vi "ziExample-HF2-RTK-PI.vi"() -> ()   [LabVIEW 2009]
doc: "This is an example for a Zurich Instruments HF2 instrument with RTK option installed. \nThis VI works together with a program for the real-time processor to implement two PI (Proportional-Integral) controllers. The controllers themselves run on the real-time processor. This VI communicates with the real-time processor to configure the controllers.\nThe program for the real-time processor is implemented in the file Main.c."
uses:
  <instrlib>/Zurich Instruments LabOne/Public/Configure/ziGetValueString.vi
  <instrlib>/Zurich Instruments LabOne/Zurich Instruments LabOne.lvlib
panel:
  in  "pid2_invert":bool
  in  "pid1_invert":bool
  in  "pid2_input_select2":enum16{"X", "Y", "R", "Theta"}(ring) caption="Signal"
  in  "pid1_input_select2":enum16{"X", "Y", "R", "Theta"}(ring) caption="Signal"
  in  "pid2_max":sgl=1.0 format="%+7.3f"
  in  "pid2_min":sgl=-1.0 caption="Range" format="%+7.3f"
  in  "pid1_max":sgl=1.0 format="%+7.3f"
  in  "pid1_min":sgl=-1.0 caption="Range" format="%+7.3f"
  in  "pid2_output_select":enum16{"Aux 1", "Aux 2", "Aux 3", "Aux 4"}(ring)=enum."Aux 2" caption="Output"
  in  "pid1_output_select":enum16{"Aux 1", "Aux 2", "Aux 3", "Aux 4"}(ring) caption="Output"
  in  "stop":bool
  out "pid2_error":dbl caption="Error" format="%_5p"
  out "pid1_error":dbl caption="Error" format="%_5p"
  in  "Port":u16=8005
  in  "Host":string="localhost"
  in  "pid2_enable":bool caption="demodOn0"
  in  "pid1_enable":bool
  in  "pid2_set_point":sgl caption="Set point" format="%+7.3f"
  in  "pid2_tc_slider":sgl(slide)=1.0 scale=0.001..10.0 scale format="%#_6p"
  in  "pid2_kp_slider":sgl(slide)=0.001 scale=0.001..1.0 scale format="%#_6p"
  in  "pid2_input_select1":T1(ring)=enum."Demod 2" caption="Demodulator"
  in  "pid1_set_point":sgl caption="Set point" format="%+7.3f"
  in  "pid1_tc_slider":sgl(slide)=1.0 scale=0.001..10.0 scale format="%#_6p"
  in  "pid1_kp_slider":sgl(slide)=0.001 scale=0.001..1.0 scale format="%#_6p"
  in  "pid1_input_select1":T1(ring) caption="Demodulator"
  # "Prop. gain"
  # "Time constant (s)"
  # "En"
  # "Inv"
  # "Tested Devices:\n- HF2LI\n\nRequires the RTK \noption"
  # "PID1"
  # "to"
  # "Prop. gain"
  # "Time constant (s)"
  # "En"
  # "Inv"
  # "PID2"
  # "to"
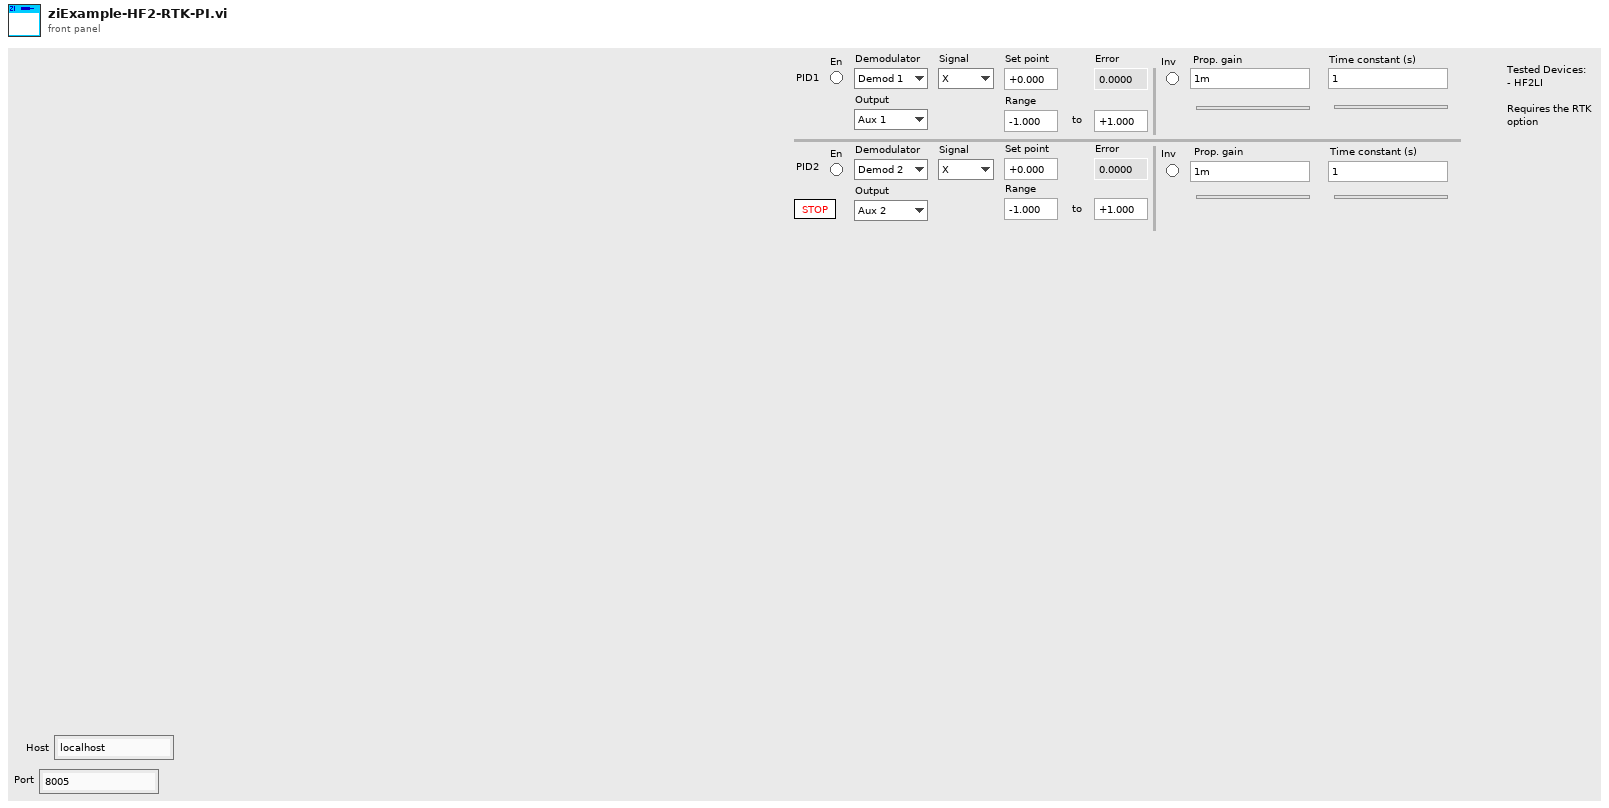
[diagram p1: front panel]
types:
  T1 = enum16{"Demod 1", "Demod 2", "Demod 3", "Demod 4", "Demod 5", "Demod 6", "Aux In 1", "Aux In 2"}
  T2 = typedef "Zurich Instruments LabOne.lvlib/ziTypeHandle.ctl" = cluster{"handleValid":bool, "Conn":u64, "Path Prefix":string, "Handle":u64, "Connected":bool, "Clockbase(s)":dbl}
  T3 = enum8{"Enabled", "Disabled", "Disabled and Grayed Out"}
  T4 = typedef "Zurich Instruments LabOne.lvlib/ziTypePollData.ctl" = cluster{"double":dbl, "Demod Sample":T5, "string":string, "Raw":u8[], "int":i32, "ScopeData":cluster{"wave":i16[], "dt (s)":dbl}, "DioInput":cluster{"Timestamp (ticks)":u64[], "Value":u32[]}, "AuxInput":cluster{"Timestamp (ticks)":u64[], "Val Ch0 (V)":dbl[], "Val Ch1 (V)":dbl[]}}
  T5 = typedef "Zurich Instruments LabOne.lvlib/ziTypeDemodSample.ctl" = cluster{"Channel":i32, "Timestamps (ticks)":u64[], "X (Vrms)":dbl[], "Y (Vrms)":dbl[], "Osc Phase (deg)":dbl[], "Freq (Hz)":dbl[], "DIO":u32[], "Aux In 0 (V)":dbl[], "Aux In 1 (V)":dbl[]}
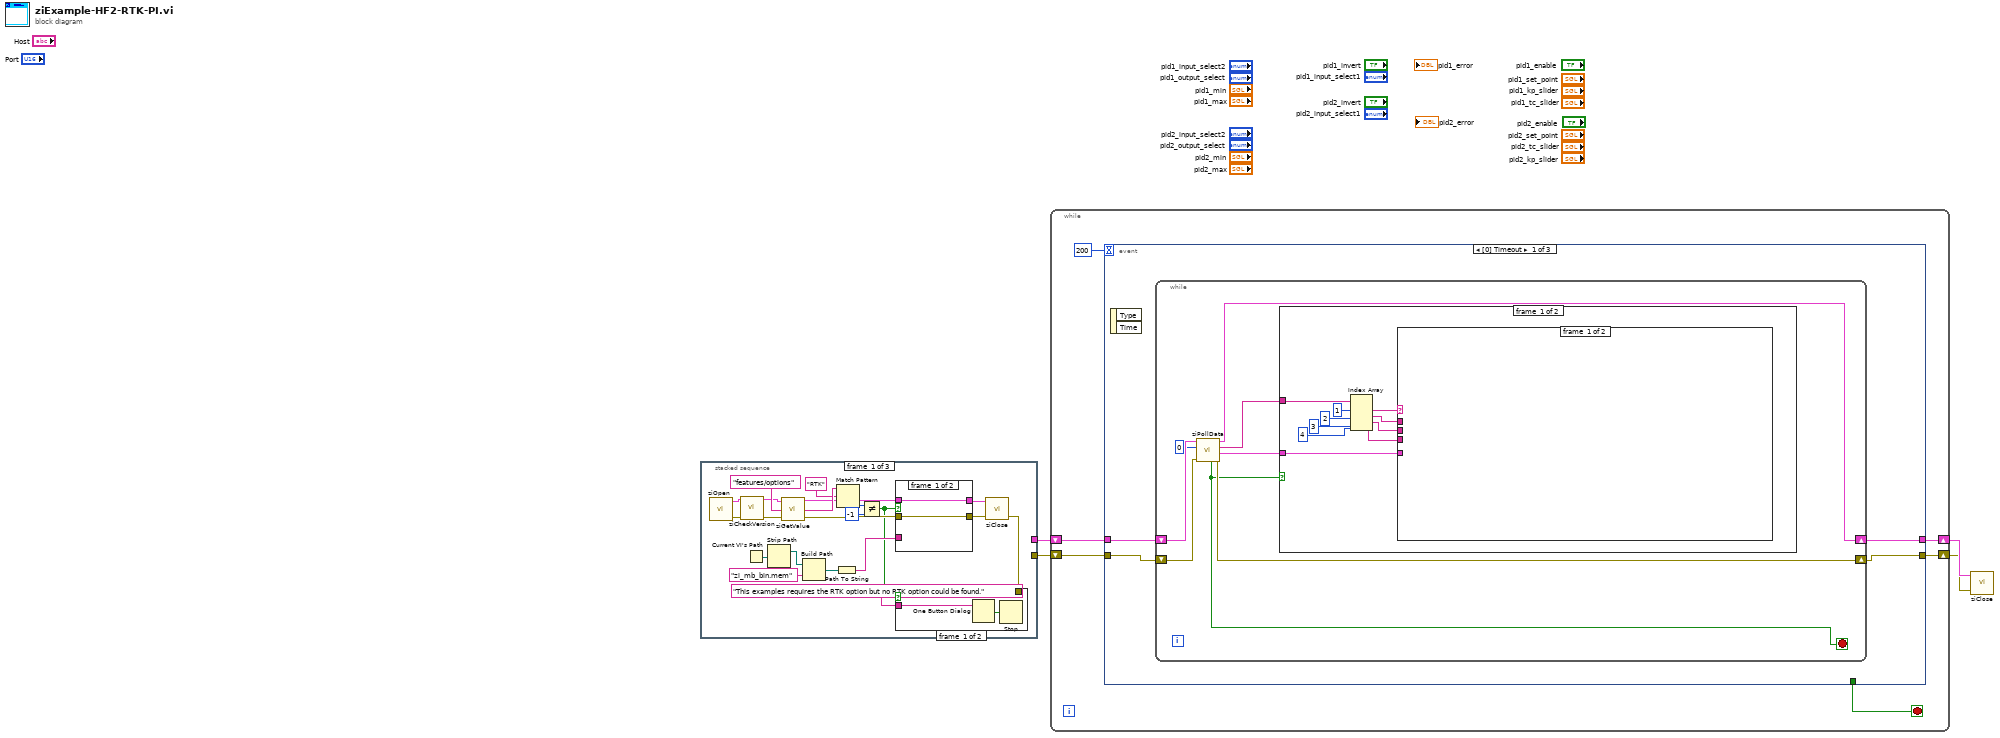
[diagram p0: block diagram]
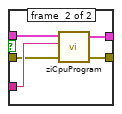
[diagram p3: hidden frame]
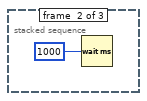
[diagram p4: hidden frame]
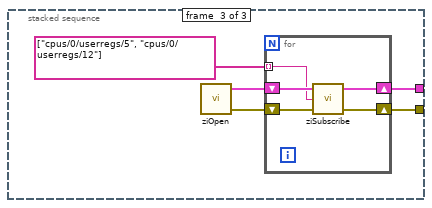
[diagram p5: hidden frame]
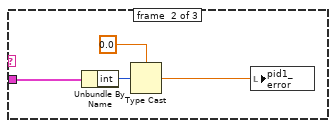
[diagram p9: hidden frame]
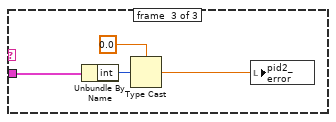
[diagram p10: hidden frame]
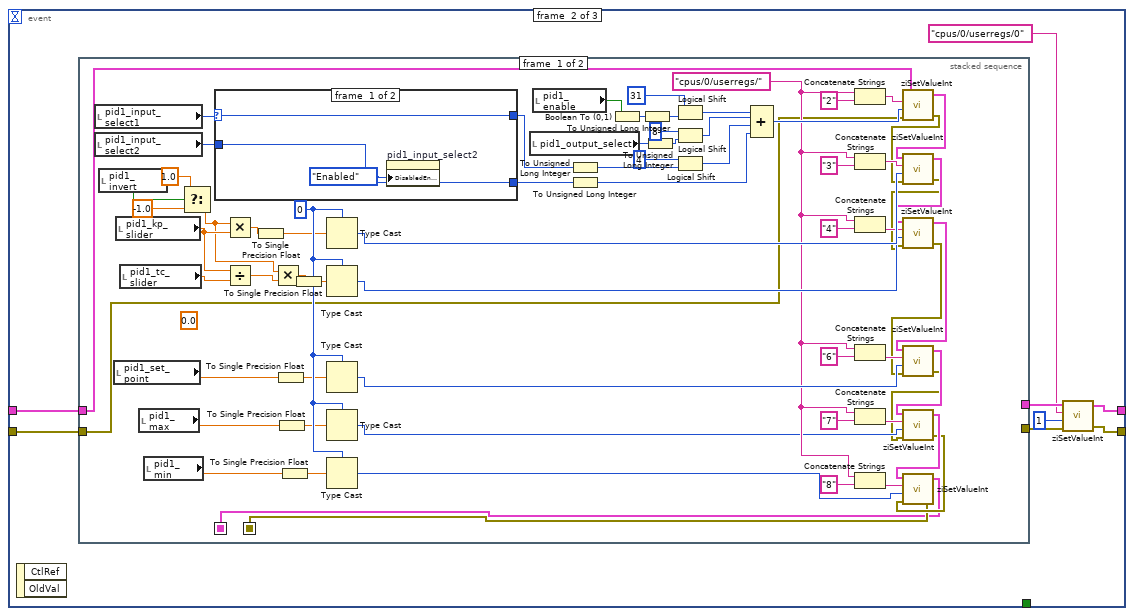
[diagram p12: hidden frame]
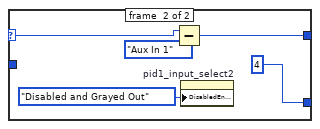
[diagram p13: hidden frame]
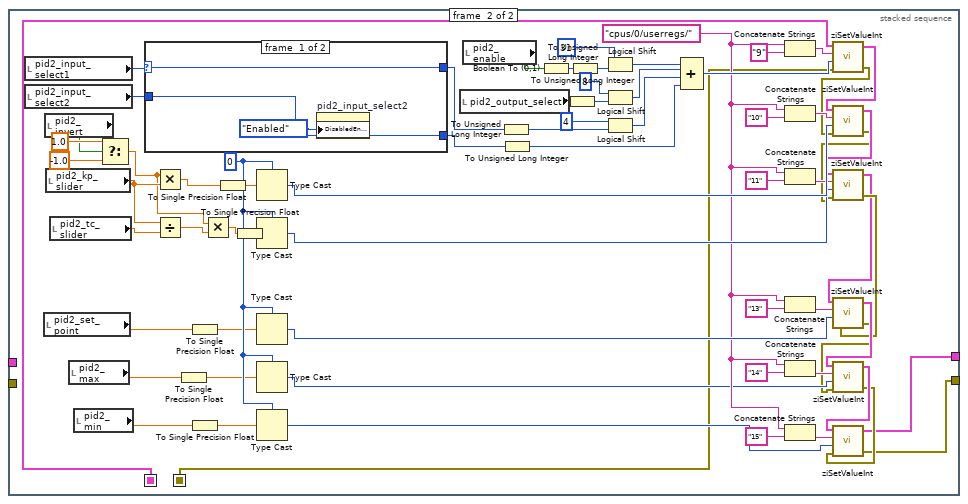
[diagram p14: hidden frame]
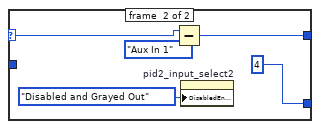
[diagram p15: hidden frame]
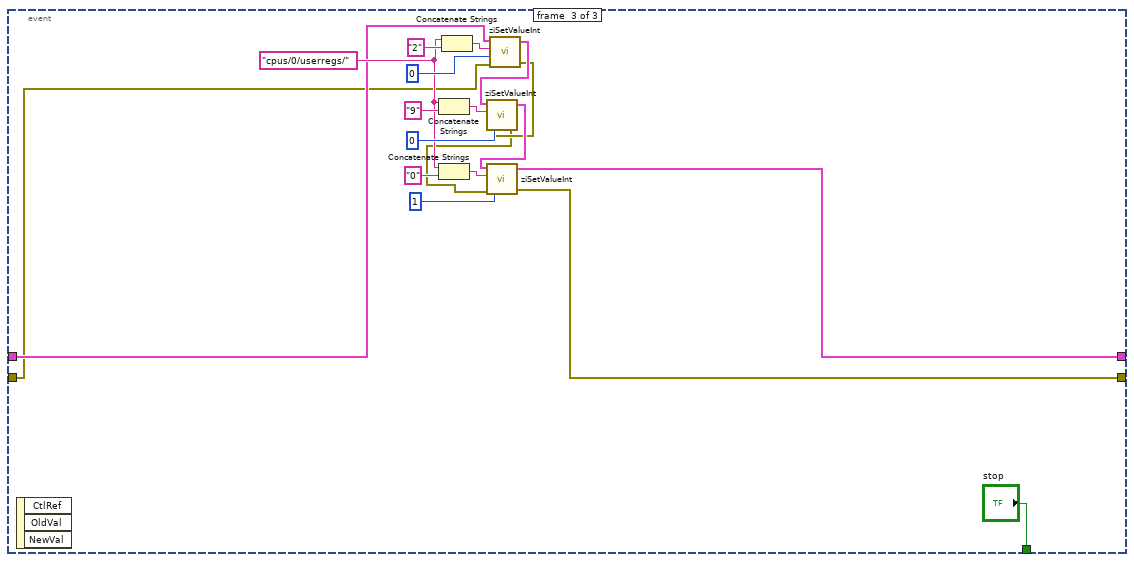
[diagram p16: hidden frame]
diagram:
  n1 = stacked-sequence {
    tunnel: [_ _ w39] -> w2
    tunnel: [_ _ w38] -> w1
    frame #0 {
      n2 = call <instrlib>:"ziOpen.vi"() -> ("Error Out"=w7:errorcluster, "HandleOut"=w8:T2)  [unwired: 4 in, 1 out]
      n3 = call <instrlib>:"ziCheckVersion.vi"("Handle In"=w8, "Error In"=w7) -> ("Handle Out"=w5:T2, "Error Out"=w6:errorcluster)  [unwired: 11 in, 1 out]
      n4 = Current VI's Path() -> (path=w20:path)
      n5 = Strip Path(path=w20) -> (stripped path=w21:path)  [unwired: 1 out]
      n6 = call-poly <instrlib>:"ziGetValue.vi"("error in"=w6, "Path"="features/options", "Handle In"=w5) -> ("error out"=w13:errorcluster, "Value"=w17:string, "Handle Out"=w12:T2)
      n7 = Build Path(base path=w21, name or relative path="zi_mb_bin.mem") -> (appended path=w19:path)
      n8 = Path To String(path=w19) -> (string=w22:string)
      n9 = Match Pattern(string=w17, regular expression="RTK" ("Path")) -> (offset past match=w15:i32)  [unwired: 1 in, 3 out]
      n10 = Not Equal?(x=w15, y=-1) -> (x != y?=w11:bool)
      n11 = case shown="False" w11 {
        tunnel: [w28 w34] -> w24
        tunnel: [w29 w33] -> w23
        tunnel: w22 -> [_ w32]
        tunnel: w13 -> [w28 w31]
        tunnel: w12 -> [w29 w30]
        frame #0 {
        }
        frame #1 {
          n12 = call <instrlib>:"ziCpuProgram.vi"("error in"=w31, "Filename"=w32, "Handle In"=w30) -> ("error out"=w34:errorcluster, "Handle Out"=w33:T2)  [unwired: 2 in]
        }
      }
      n13 = call <instrlib>:"ziClose.vi"("Error In"=w24, "Handle In"=w23) -> ("Error Out"=w10:errorcluster)  [unwired: 3 out]
      n14 = case shown="False" w11 {
        tunnel: w10 -> [_ _]
        tunnel: "This examples requires the RTK option but no RTK option could be found." ("message") -> [w26 _]
        frame #0 {
          n15 = One Button Dialog(message=w26) -> (true=w27:bool)  [unwired: 1 in]
          n16 = Stop(stop? (T)=w27) -> ()
        }
        frame #1 {
        }
      }
    }
    frame #1 {
      n17 = Wait (ms)(milliseconds to wait=u32 1000) -> ()  [unwired: 1 out]
    }
    frame #2 {
      n18 = call <instrlib>:"ziOpen.vi"() -> ("Error Out"=w36:errorcluster, "HandleOut"=w37:T2)  [unwired: 4 in, 1 out]
      n19 = for {
        shift-right: [w43] -> w39
        shift-left: w37 -> [w45]
        shift-right: [w42] -> w38
        shift-left: w36 -> [w44]
        tunnel: string[] ["cpus/0/userregs/5", "cpus/0/userregs/12"] -> [w41] mode=indexing
        n20 = call <instrlib>:"ziSubscribe.vi"("error in"=w44, "Path ()"=w41, "Handle In"=w45) -> ("error out"=w42:errorcluster, "Handle Out"=w43:T2)  [unwired: 1 in]
      }
    }
  }
  n21 = while {
    shift-right: [w49] -> w4
    shift-left: w2 -> [w51]
    shift-right: [w48] -> w3
    shift-left: w1 -> [w50]
    stop <- w47 stop-if-true
    n22 = event shown="[0] Timeout" {
      selector: _ -> [_ _ _]
      dyn-events: _ -> [_ _ _]
      timeout: 200 -> [_ _ _]
      tunnel: w51 -> [w55 w98 w258]
      tunnel: w50 -> [w54 w97 w254]
      tunnel: [w53 w95 w257] -> w49
      tunnel: [w52 w96 w251] -> w48
      tunnel: [_ _ "stop"] -> w47
      event #0 {
        n23 = event-data() -> ()  [unwired: 3 out]
        n24 = while {
          shift-right: [w61] -> w53
          shift-left: w55 -> [w63]
          shift-right: [w60] -> w52
          shift-left: w54 -> [w62]
          stop <- w59 stop-if-true
          n25 = call <instrlib>:"ziPollData.vi"("Error In"=w62, "TimeOut ms (50)"=0, "Handle In"=w63) -> ("Error Out"=w60:errorcluster, "Data Out"=w57:T4, "PathArray"=w58:string[], "Handle Out"=w61:T2, "Timed Out"=w59:bool)  [unwired: 3 in, 1 out]
          n26 = case shown="False" w59 {
            tunnel: w58 -> [w73 _]
            tunnel: w57 -> [w68 _]
            frame #0 {
              n27 = Index Array(array=w73, index #1=1 ("index"), index #2=2 ("index"), index #3=3 ("index"), index #4=4 ("index")) -> (element #1=w71:string, element #2=w69:string, element #3=w66:string, element #4=w64:string)
              n28 = case shown="\"CPUS\"" w71 {
                tunnel: w69 -> [_ w77]
                tunnel: w68 -> [_ w75]
                tunnel: w66 -> [_ w76]
                tunnel: w64 -> [_ w74]
                frame #0 {
                }
                frame #1 {
                  n29 = case shown="\"0\"" w77 {
                    tunnel: w76 -> [_ w80]
                    tunnel: w75 -> [_ w79]
                    tunnel: w74 -> [_ w78]
                    frame #0 {
                    }
                    frame #1 {
                      n30 = case shown="\"USERREGS\"" w80 {
                        tunnel: w79 -> [_ w81]
                        tunnel: w78 -> [_ w82]
                        frame #0 {
                        }
                        frame #1 {
                          n31 = case shown="\"5\"" w82 {
                            tunnel: w81 -> [_ w86 w90]
                            frame #0 {
                            }
                            frame #1 {
                              n32 = Unbundle By Name(w86) -> ("int"=w85:i32)
                              n33 = Type Cast(type=sgl 0.0, x=w85) -> (*(type *) &x=w83:sgl)
                              n34 = local write "pid1_error"(w83) -> ()
                            }
                            frame #2 {
                              n35 = Unbundle By Name(w90) -> ("int"=w89:i32)
                              n36 = Type Cast(type=sgl 0.0, x=w89) -> (*(type *) &x=w87:sgl)
                              n37 = local write "pid2_error"(w87) -> ()
                            }
                          }
                        }
                      }
                    }
                  }
                }
              }
            }
            frame #1 {
            }
          }
        }
      }
      event #1 {
        n38 = event-data() -> ()  [unwired: 3 out]
        n39 = stacked-sequence {
          seq-local: [w117 _] -> [_ w195]
          seq-local: [w118 _] -> [_ w194]
          tunnel: w98 -> [w128 _]
          tunnel: w97 -> [w127 _]
          tunnel: [_ w197] -> w93
          tunnel: [_ w196] -> w94
          frame #0 {
            w138 = 0
            w131 = "cpus/0/userregs/"
            (unwired) sgl 0.0 ("number")
            n40 = local read "pid1_input_select1"() -> (w164:T1)
            n41 = local read "pid1_input_select2"() -> (w163:enum16{"X", "Y", "R", "Theta"})
            n42 = local read "pid1_invert"() -> (w108:bool)
            n43 = local read "pid1_set_point"() -> (w142:sgl)
            n44 = local read "pid1_kp_slider"() -> (w166:sgl)
            n45 = local read "pid1_tc_slider"() -> (w165:sgl)
            n46 = local read "pid1_max"() -> (w137:sgl)
            n47 = local read "pid1_min"() -> (w136:sgl)
            n48 = Select(t=1.0, s=w108, f=-1.0) -> (s? t:f=w104:dbl)
            n49 = case shown="\"Aux In 1\", \"Aux In 2\"" w164 {
              selector: w164 -> [w169 w174]
              tunnel: [w169 w172] -> w156
              tunnel: [w168 4] -> w155
              tunnel: w163 -> [w168 _]
              frame #0 {
                n50 = property on="pid1_input_select2" class="Enum (strict)"("DisabledEnum"=T3."Enabled" ("Disabled")) -> ()  [unwired: 2 in, 2 out]
              }
              frame #1 {
                n51 = Subtract(x=w174, y=T1."Aux In 1") -> (x-y=w172:u16)
                n52 = property on="pid1_input_select2" class="Enum (strict)"("DisabledEnum"=T3."Disabled and Grayed Out" ("Disabled")) -> ()  [unwired: 2 in, 2 out]
              }
            }
            n53 = Multiply(x=w104, y=w166) -> (x*y=w148:dbl)
            n54 = Divide(x=w166, y=w165) -> (x/y=w105:sgl)
            n55 = To Single Precision Float(number=w148) -> (single precision float=w103:sgl)
            n56 = Multiply(x=w104, y=w105) -> (x*y=w146:dbl)
            n57 = To Single Precision Float(number=w142) -> (single precision float=w101:sgl)
            n58 = To Single Precision Float(number=w137) -> (single precision float=w100:sgl)
            n59 = To Single Precision Float(number=w136) -> (single precision float=w99:sgl)
            n60 = To Single Precision Float(number=w146) -> (single precision float=w102:sgl)
            n61 = Type Cast(type=w138, x=w103) -> (*(type *) &x=w147:i32)
            n62 = Type Cast(type=w138, x=w102) -> (*(type *) &x=w143:i32)
            n63 = Type Cast(type=w138, x=w101) -> (*(type *) &x=w139:i32)
            n64 = Type Cast(type=w138, x=w100) -> (*(type *) &x=w129:i32)
            n65 = Type Cast(type=w138, x=w99) -> (*(type *) &x=w130:i32)
            n66 = local read "pid1_output_select"() -> (w151:enum16{"Aux 1", "Aux 2", "Aux 3", "Aux 4"})
            n67 = local read "pid1_enable"() -> (w162:bool)
            n68 = To Unsigned Long Integer(number=w156) -> (unsigned 32bit integer=w115:u32)
            n69 = To Unsigned Long Integer(number=w155) -> (unsigned 32bit integer=w112:u32)
            n70 = Boolean To (0,1)(Boolean=w162) -> (0, 1=w160:i16)
            n71 = To Unsigned Long Integer(number=w160) -> (unsigned 32bit integer=w116:u32)
            n72 = To Unsigned Long Integer(number=w151) -> (unsigned 32bit integer=w114:u32)
            n73 = Logical Shift(y=u32 31, x=w116) -> (x << y=w158:u32)
            n74 = Logical Shift(y=u32 8, x=w114) -> (x << y=w113:u32)
            n75 = Logical Shift(y=u32 4, x=w115) -> (x << y=w111:u32)
            n76 = Compound Arithmetic op=ADD(w158, w113, w111, w112) -> (w161:u32)
            n77 = Concatenate Strings(w131, "2" ("string")) -> (w154:string)
            n78 = Concatenate Strings(w131, "3" ("string")) -> (w150:string)
            n79 = Concatenate Strings(w131, "4" ("string")) -> (w145:string)
            n80 = Concatenate Strings(w131, "6" ("string")) -> (w141:string)
            n81 = Concatenate Strings(w131, "7" ("string")) -> (w134:string)
            n82 = Concatenate Strings(w131, "8" ("string")) -> (w133:string)
            n83 = call <instrlib>:"ziSetValueInt.vi"("Error in"=w127, "Value"=w161, "Path"=w154, "Handle in"=w128) -> ("Error out"=w122:errorcluster, "Handle out"=w126:T2)  [unwired: 1 in]
            n84 = call <instrlib>:"ziSetValueInt.vi"("Error in"=w122, "Value"=w147, "Path"=w150, "Handle in"=w126) -> ("Error out"=w121:errorcluster, "Handle out"=w125:T2)  [unwired: 1 in]
            n85 = call <instrlib>:"ziSetValueInt.vi"("Error in"=w121, "Value"=w143, "Path"=w145, "Handle in"=w125) -> ("Error out"=w110:errorcluster, "Handle out"=w109:T2)  [unwired: 1 in]
            n86 = call <instrlib>:"ziSetValueInt.vi"("Error in"=w110, "Value"=w139, "Path"=w141, "Handle in"=w109) -> ("Error out"=w120:errorcluster, "Handle out"=w124:T2)  [unwired: 1 in]
            n87 = call <instrlib>:"ziSetValueInt.vi"("Error in"=w120, "Value"=w129, "Path"=w134, "Handle in"=w124) -> ("Error out"=w119:errorcluster, "Handle out"=w123:T2)  [unwired: 1 in]
            n88 = call <instrlib>:"ziSetValueInt.vi"("Error in"=w119, "Value"=w130, "Path"=w133, "Handle in"=w123) -> ("Error out"=w118:errorcluster, "Handle out"=w117:T2)  [unwired: 1 in]
          }
          frame #1 {
            w215 = 0
            w208 = "cpus/0/userregs/"
            n89 = local read "pid2_input_select1"() -> (w240:T1)
            n90 = local read "pid2_input_select2"() -> (w239:enum16{"X", "Y", "R", "Theta"})
            n91 = local read "pid2_set_point"() -> (w219:sgl)
            n92 = local read "pid2_invert"() -> (w180:bool)
            n93 = local read "pid2_kp_slider"() -> (w242:sgl)
            n94 = local read "pid2_tc_slider"() -> (w241:sgl)
            n95 = local read "pid2_max"() -> (w214:sgl)
            n96 = local read "pid2_min"() -> (w213:sgl)
            n97 = Select(t=1.0, s=w180, f=-1.0) -> (s? t:f=w183:dbl)
            n98 = case shown="\"Aux In 1\", \"Aux In 2\"" w240 {
              selector: w240 -> [w245 w250]
              tunnel: [w245 w248] -> w232
              tunnel: [w244 4] -> w190
              tunnel: w239 -> [w244 _]
              frame #0 {
                n99 = property on="pid2_input_select2" class="Enum (strict)"("DisabledEnum"=T3."Enabled" ("Disabled")) -> ()  [unwired: 2 in, 2 out]
              }
              frame #1 {
                n100 = Subtract(x=w250, y=T1."Aux In 1") -> (x-y=w248:u16)
                n101 = property on="pid2_input_select2" class="Enum (strict)"("DisabledEnum"=T3."Disabled and Grayed Out" ("Disabled")) -> ()  [unwired: 2 in, 2 out]
              }
            }
            n102 = Multiply(x=w183, y=w242) -> (x*y=w225:dbl)
            n103 = Divide(x=w242, y=w241) -> (x/y=w184:sgl)
            n104 = To Single Precision Float(number=w214) -> (single precision float=w176:sgl)
            n105 = To Single Precision Float(number=w219) -> (single precision float=w177:sgl)
            n106 = To Single Precision Float(number=w213) -> (single precision float=w175:sgl)
            n107 = Multiply(x=w183, y=w184) -> (x*y=w223:dbl)
            n108 = To Single Precision Float(number=w225) -> (single precision float=w179:sgl)
            n109 = To Single Precision Float(number=w223) -> (single precision float=w178:sgl)
            n110 = Type Cast(type=w215, x=w179) -> (*(type *) &x=w224:i32)
            n111 = Type Cast(type=w215, x=w178) -> (*(type *) &x=w220:i32)
            n112 = Type Cast(type=w215, x=w177) -> (*(type *) &x=w216:i32)
            n113 = Type Cast(type=w215, x=w176) -> (*(type *) &x=w206:i32)
            n114 = Type Cast(type=w215, x=w175) -> (*(type *) &x=w207:i32)
            n115 = local read "pid2_output_select"() -> (w228:enum16{"Aux 1", "Aux 2", "Aux 3", "Aux 4"})
            n116 = local read "pid2_enable"() -> (w238:bool)
            n117 = To Unsigned Long Integer(number=w232) -> (unsigned 32bit integer=w188:u32)
            n118 = To Unsigned Long Integer(number=w190) -> (unsigned 32bit integer=w187:u32)
            n119 = Boolean To (0,1)(Boolean=w238) -> (0, 1=w236:i16)
            n120 = To Unsigned Long Integer(number=w228) -> (unsigned 32bit integer=w192:u32)
            n121 = To Unsigned Long Integer(number=w236) -> (unsigned 32bit integer=w193:u32)
            n122 = Logical Shift(y=i8 31, x=w193) -> (x << y=w234:u32)
            n123 = Logical Shift(y=i16 8, x=w192) -> (x << y=w191:u32)
            n124 = Logical Shift(y=i16 4, x=w188) -> (x << y=w189:u32)
            n125 = Compound Arithmetic op=ADD(w234, w191, w189, w187) -> (w237:u32)
            n126 = Concatenate Strings(w208, "9" ("string")) -> (w231:string)
            n127 = Concatenate Strings(w208, "10" ("string")) -> (w227:string)
            n128 = Concatenate Strings(w208, "11" ("string")) -> (w222:string)
            n129 = Concatenate Strings(w208, "13" ("string")) -> (w218:string)
            n130 = Concatenate Strings(w208, "14" ("string")) -> (w211:string)
            n131 = Concatenate Strings(w208, "15" ("string")) -> (w210:string)
            n132 = call <instrlib>:"ziSetValueInt.vi"("Error in"=w194, "Value"=w237, "Path"=w231, "Handle in"=w195) -> ("Error out"=w201:errorcluster, "Handle out"=w205:T2)  [unwired: 1 in]
            n133 = call <instrlib>:"ziSetValueInt.vi"("Error in"=w201, "Value"=w224, "Path"=w227, "Handle in"=w205) -> ("Error out"=w200:errorcluster, "Handle out"=w204:T2)  [unwired: 1 in]
            n134 = call <instrlib>:"ziSetValueInt.vi"("Error in"=w200, "Value"=w220, "Path"=w222, "Handle in"=w204) -> ("Error out"=w186:errorcluster, "Handle out"=w185:T2)  [unwired: 1 in]
            n135 = call <instrlib>:"ziSetValueInt.vi"("Error in"=w186, "Value"=w216, "Path"=w218, "Handle in"=w185) -> ("Error out"=w199:errorcluster, "Handle out"=w203:T2)  [unwired: 1 in]
            n136 = call <instrlib>:"ziSetValueInt.vi"("Error in"=w199, "Value"=w206, "Path"=w211, "Handle in"=w203) -> ("Error out"=w198:errorcluster, "Handle out"=w202:T2)  [unwired: 1 in]
            n137 = call <instrlib>:"ziSetValueInt.vi"("Error in"=w198, "Value"=w207, "Path"=w210, "Handle in"=w202) -> ("Error out"=w196:errorcluster, "Handle out"=w197:T2)  [unwired: 1 in]
          }
        }
        n138 = call <instrlib>:"ziSetValueInt.vi"("Error in"=w94, "Value"=i64 1, "Path"="cpus/0/userregs/0", "Handle in"=w93) -> ("Error out"=w96:errorcluster, "Handle out"=w95:T2)  [unwired: 1 in]
      }
      event #2 {
        w260 = "cpus/0/userregs/"
        n139 = event-data() -> ()  [unwired: 4 out]
        n140 = Concatenate Strings(w260, "9" ("string")) -> (w266:string)
        n141 = Concatenate Strings(w260, "0" ("string")) -> (w262:string)
        n142 = Concatenate Strings(w260, "2" ("string")) -> (w267:string)
        n143 = call <instrlib>:"ziSetValueInt.vi"("Error in"=w254, "Value"=i64 0, "Path"=w267, "Handle in"=w258) -> ("Error out"=w253:errorcluster, "Handle out"=w255:T2)  [unwired: 1 in]
        n144 = call <instrlib>:"ziSetValueInt.vi"("Error in"=w253, "Value"=i64 0, "Path"=w266, "Handle in"=w255) -> ("Error out"=w252:errorcluster, "Handle out"=w256:T2)  [unwired: 1 in]
        n145 = call <instrlib>:"ziSetValueInt.vi"("Error in"=w252, "Value"=i64 1, "Path"=w262, "Handle in"=w256) -> ("Error out"=w251:errorcluster, "Handle out"=w257:T2)  [unwired: 1 in]
      }
    }
  }
  n146 = call <instrlib>:"ziClose.vi"("Error In"=w3, "Handle In"=w4) -> ()  [unwired: 4 out]
